vi "统计行数.vi"(10 "测试时间":string) -> (3 "Rows Fetched":i32)   [LabVIEW 2014]
panel:
  out "Data":string[][](array[string])
  out "error out":errorcluster
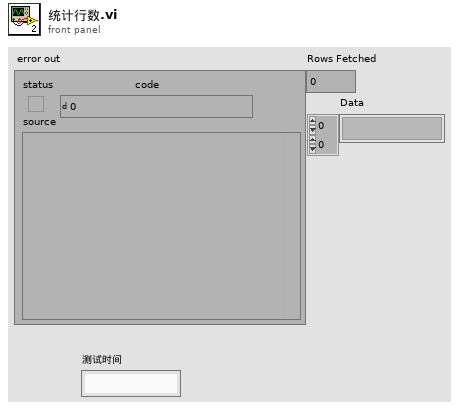
[diagram p1: front panel]
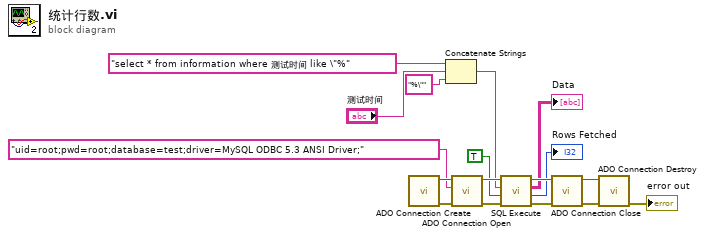
[diagram p0: block diagram]
diagram:
  n1 = call "ADO Connection Create.vi"() -> ("error out"=w16:errorcluster, "ADODB._Connection Out"=w17:refnum<k7>)  [unwired: 10 in]
  n2 = Concatenate Strings("select * from information where 测试时间 like \"%" ("Command Text"), "测试时间", "%\"" ("Command Text")) -> (w1:string)
  n3 = call "ADO Connection Open.vi"("error in (no error)"=w16, "ConnectionString"="uid=root;pwd=root;database=test;driver=MySQL ODBC 5.3 ANSI Driver;", "ADODB._Connection In"=w17) -> ("error out"=w14:errorcluster, "ADODB._Connection Out"=w15:refnum<k7>)  [unwired: 7 in]
  n4 = call "SQL Execute.vi"("error in (no error)"=w14, "Return Data (T)"=TRUE, "Command Text"=w1, "ADODB._Connection In"=w15) -> ("error out"=w12:errorcluster, "Rows Fetched"=→"Rows Fetched":i32, "Data"=→"Data":string[][], "ADODB._Connection Out"=w13:refnum<k7>)  [unwired: 4 in]
  n5 = call "ADO Connection Close.vi"("error in (no error)"=w12, "ADODB._Connection In"=w13) -> ("error out"=w10:errorcluster, "ADODB._Connection Out"=w11:refnum<k7>)  [unwired: 8 in]
  n6 = call "ADO Connection Destroy.vi"("error in (no error)"=w10, "ADODB._Connection In"=w11) -> ("error out"=→"error out":errorcluster)  [unwired: 9 in]
